vi "Send Report Error.vi"(7 "Priority":T1=enum."Normal" caption="Message Priority (Normal)", 8 "error in (no error)":errorcluster, 9 "Stopped by the Caller?":bool, 10 "Caller Error Handler":refnum<class "Iterator Report Error Msg.lvclass">, 11 "Caller Enqueuer in":refnum<class "Message Enqueuer.lvclass">) -> (0 "error out":errorcluster, 3 "Caller Enqueuer out":refnum<class "Message Enqueuer.lvclass">)   [LabVIEW 2017, in "Iterator Actor.lvlib" / "Iterator Report Error Msg.lvclass"]
doc: "Sends the <b>Iterator Actor 2.lvlib:Stop Iterate Msg.lvclass</b> message.\n\nThis message will call <b>Stop Iterate.vi</b> on the <b>Iterator Actor 2.lvlib:Iterator Actor 2.lvclass</b> actor.\n\n<b>Stop Iterate.vi Description</b>"
uses:
  Iterator Report Error Msg.lvclass
  <vilib>/ActorFramework/Message Enqueuer/Message Enqueuer.lvclass
  <vilib>/ActorFramework/Message Enqueuer/Message Priority.ctl
  C:/Program Files (x86)/National Instruments/LabVIEW 2017/vi.lib/ActorFramework/Message/Message.lvclass
  Iterator Report Error Msg.lvclass/Iterator Report Error Msg.ctl
  <vilib>/ActorFramework/Message Enqueuer/Message Enqueuer.lvclass/Message Enqueuer.ctl
  <vilib>/ActorFramework/Message Priority Queue/Priority Enqueue.vi
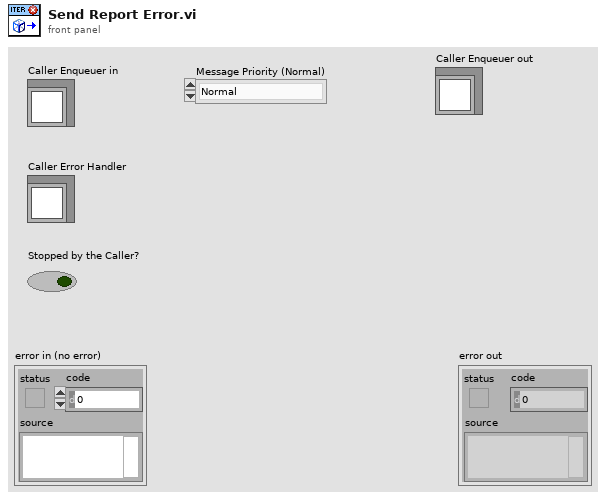
[diagram p1: front panel]
types:
  T1 = typedef "Actor Framework.lvlib/Message Enqueuer.lvclass/Message Priority.ctl" = enum16{"Low", "Normal", "High"}
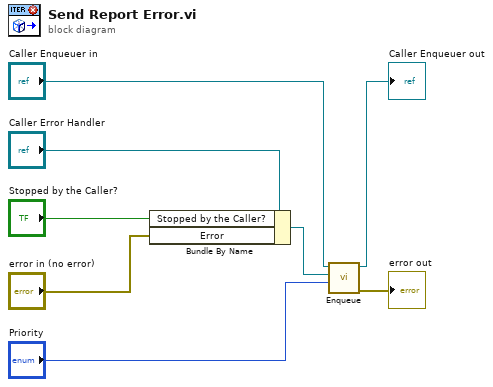
[diagram p0: block diagram]
diagram:
  n1 = Bundle By Name(cluster="Caller Error Handler", "Stopped by the Caller?"="Stopped by the Caller?", "Error"="error in (no error)") -> (w3:refnum<class "Iterator Report Error Msg.lvclass">)
  n2 = call <vilib>:"Enqueue.vi"("Message Priority (Normal)"="Priority", "Message"=w3, "Message Enqueuer in"="Caller Enqueuer in") -> ("error out"=→"error out":errorcluster, "Message Enqueuer out"=→"Caller Enqueuer out":refnum<class "Message Enqueuer.lvclass">)  [unwired: 7 in]
